vi "FourCornerAntennaAlignment.vi"(10 "Y corners, 1, 8, 57, 64":dbl[](array[numeric])=[144.21, 145.21, 338.21, 339.2] format="%.4f", 11 "X corners, 1, 8, 57, 64":dbl[](array[numeric])=[204.42, 398.3, 203.44, 397.44] format="%.4f") -> (1 "x angle all":dbl, 3 "x direction angle":dbl format="%.4f")   [LabVIEW 2017]
doc: "uses motion controller coordinates of the four corner crosshairs of the antenna to compute the angle that the antenna is rotated wrt to the x y axes of the motion system."
uses:
  <vilib>/Analysis/baseanly.llb/Mean (DBL).vi
  <vilib>/Analysis/NI_AALBase.lvlib
panel:
  out "degrees 2":dbl[](array[numeric])
  out "standard deviation":dbl format="%.5f"
  out "y direction angle":dbl format="%.4f"
  out "degrees":dbl[](array[numeric])
  # "could drop points outside the sdev\n\nor\n\ntake the two x direction computations - doing this for now"
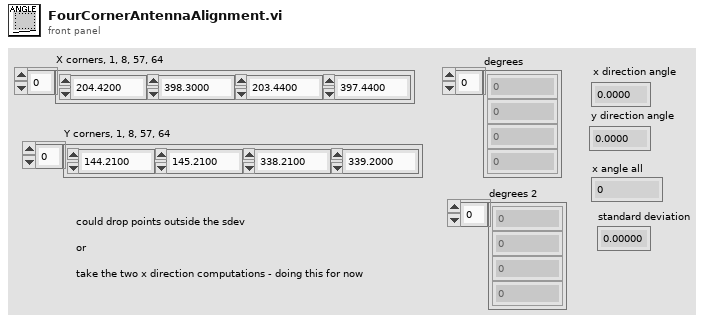
[diagram p1: front panel]
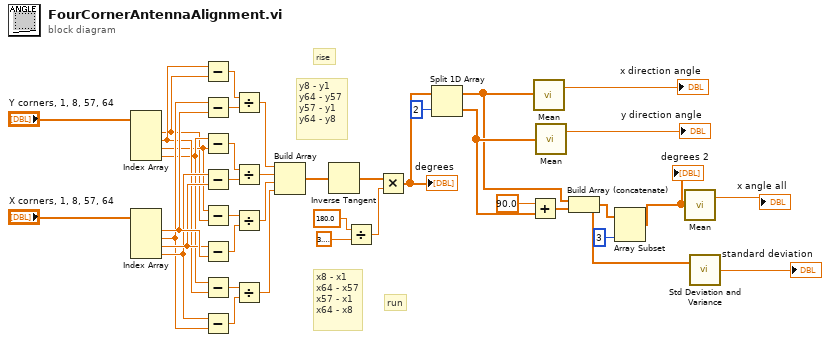
[diagram p0: block diagram]
diagram:
  # "y8 - y1\ny64 - y57\ny57 - y1\ny64 - y8"
  # "x8 - x1\nx64 - x57\nx57 - x1\nx64 - x8"
  # "rise"
  # "run"
  n1 = Index Array(array="Y corners, 1, 8, 57, 64") -> (element #1=w26:dbl, element #2=w29:dbl, element #3=w27:dbl, element #4=w28:dbl)  [unwired: 4 in]
  n2 = Index Array(array="X corners, 1, 8, 57, 64") -> (element #1=w33:dbl, element #2=w30:dbl, element #3=w32:dbl, element #4=w31:dbl)  [unwired: 4 in]
  n3 = Subtract(x=w29, y=w26) -> (x-y=w24:dbl)
  n4 = Subtract(x=w30, y=w33) -> (x-y=w39:dbl)
  n5 = Subtract(x=w28, y=w27) -> (x-y=w23:dbl)
  n6 = Subtract(x=w31, y=w32) -> (x-y=w38:dbl)
  n7 = Subtract(x=w27, y=w26) -> (x-y=w21:dbl)
  n8 = Subtract(x=w32, y=w33) -> (x-y=w22:dbl)
  n9 = Subtract(x=w28, y=w29) -> (x-y=w20:dbl)
  n10 = Subtract(x=w31, y=w30) -> (x-y=w19:dbl)
  n11 = Divide(x=w24, y=w39) -> (x/y=w18:dbl)
  n12 = Divide(x=w23, y=w38) -> (x/y=w17:dbl)
  n13 = Divide(x=w21, y=w22) -> (x/y=w16:dbl)
  n14 = Divide(x=w20, y=w19) -> (x/y=w15:dbl)
  n15 = Build Array(w18, w17, w16, w15) -> (w14:dbl[])
  n16 = Inverse Tangent(1:w14) -> (0:w34:dbl[])
  n17 = Divide(x=180.0 ("y"), y=3.141592653589793) -> (x/y=w37:dbl)
  n18 = Multiply(x=w34, y=w37) -> (x*y=w13:dbl[])
  "degrees" <- w13
  n19 = Split 1D Array(array=w13, index=2) -> (first subarray=w6:dbl[], second subarray=w8:dbl[])
  n20 = Add(x=90.0, y=w8) -> (x+y=w7:dbl[])
  n21 = call-poly <vilib>:"Mean.vi"("X"=w6) -> ("mean"=→"x direction angle":dbl)  [unwired: 1 out]
  n22 = call-poly <vilib>:"Mean.vi"("X"=w8) -> ("mean"=→"y direction angle":dbl)  [unwired: 1 out]
  n23 = Build Array (concatenate)(w6, w7) -> (w3:dbl[])
  n24 = Array Subset(array=w3, length=3) -> (w1:dbl[])  [unwired: 1 in]
  "degrees 2" <- w1
  n25 = call-poly <vilib>:"Mean.vi"("X"=w1) -> ("mean"=→"x angle all":dbl)  [unwired: 1 out]
  n26 = call <vilib>:"Std Deviation and Variance.vi"("X"=w3) -> ("standard deviation"=→"standard deviation":dbl)  [unwired: 1 in, 2 out]
